vi "Encoder_VI.vi"() -> ()   [LabVIEW 2016]
uses:
  Control 1.ctl
  <vilib>/Instr/_visa.llb/VISA Flush IO Buffer Mask.ctl
  <vilib>/Instr/_visa.llb/VISA Configure Serial Port (Instr).vi
  <vilib>/Utility/file.llb/Write Delimited Spreadsheet (string).vi
panel:
  out "Serial Settings:Number of Bytes at Serial Port":u32
  out "ERRO":dbl
  in  "Limpar":bool
  out "Waveform Graph":waveform(i32)(graph)
  out "Pulso\nInstantâneo":i32
  out "Tempo\nInstantâneo (ms)":u32
  out "iniicio":u32
  in  "Cronômetro para início (s)":string
  out "Identificação":u32
  in  "Endereço":string
  in  "stop":bool
  out "start read":bool
  out "save":bool
  out "start device":bool
  in  "Parar":bool
  out "Configurado Man":bool
  out "Configurado Auto":bool
  out "Desconectado":bool
  out "Conectado":bool
  in  "Frequência \nManual (Hz)":i16
  in  "Frequência \nAutomática (Hz)":u8(ring) items=["50", "100", "200", "500", "1000"]
  in  "Leitura Automática":bool
  in  "Conectar":bool
  in  "salvar dados":bool
  in  "Iniciar dispositivo":bool
  in  "Inicia auto":bool
  in  "Configurar":bool
  in  "Identificar":bool
  in  "Codificar":bool
  out "?":string
  in  "Serial":refnum<visa-resource-name>
  # "Leitura de Encoder - CEFISE"
  # "Status"
  # "Resultado da medida"
  # "Leitura Manual"
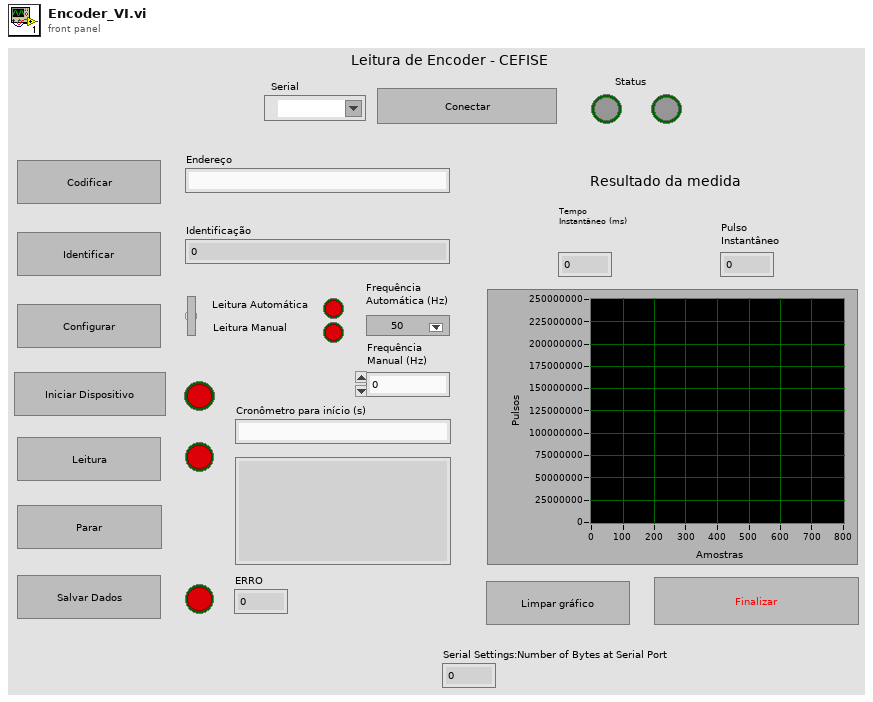
[diagram p1: front panel]
types:
  T1 = typedef "Control 1.ctl" = enum16{"Init", "Wait", "Id", "Codificacao", "Config. Auto", "Config. Man", "Start device", "Read Auto", "Read Again", "Read First", "Stop device", "End", "Save", "erro", "Plot", "Organize", "Limpa"}
  T2 = enum8{"Enabled", "Disabled", "Disabled and Grayed Out"}
  T3 = typedef "VISA Flush IO Buffer Mask.ctl" = u16
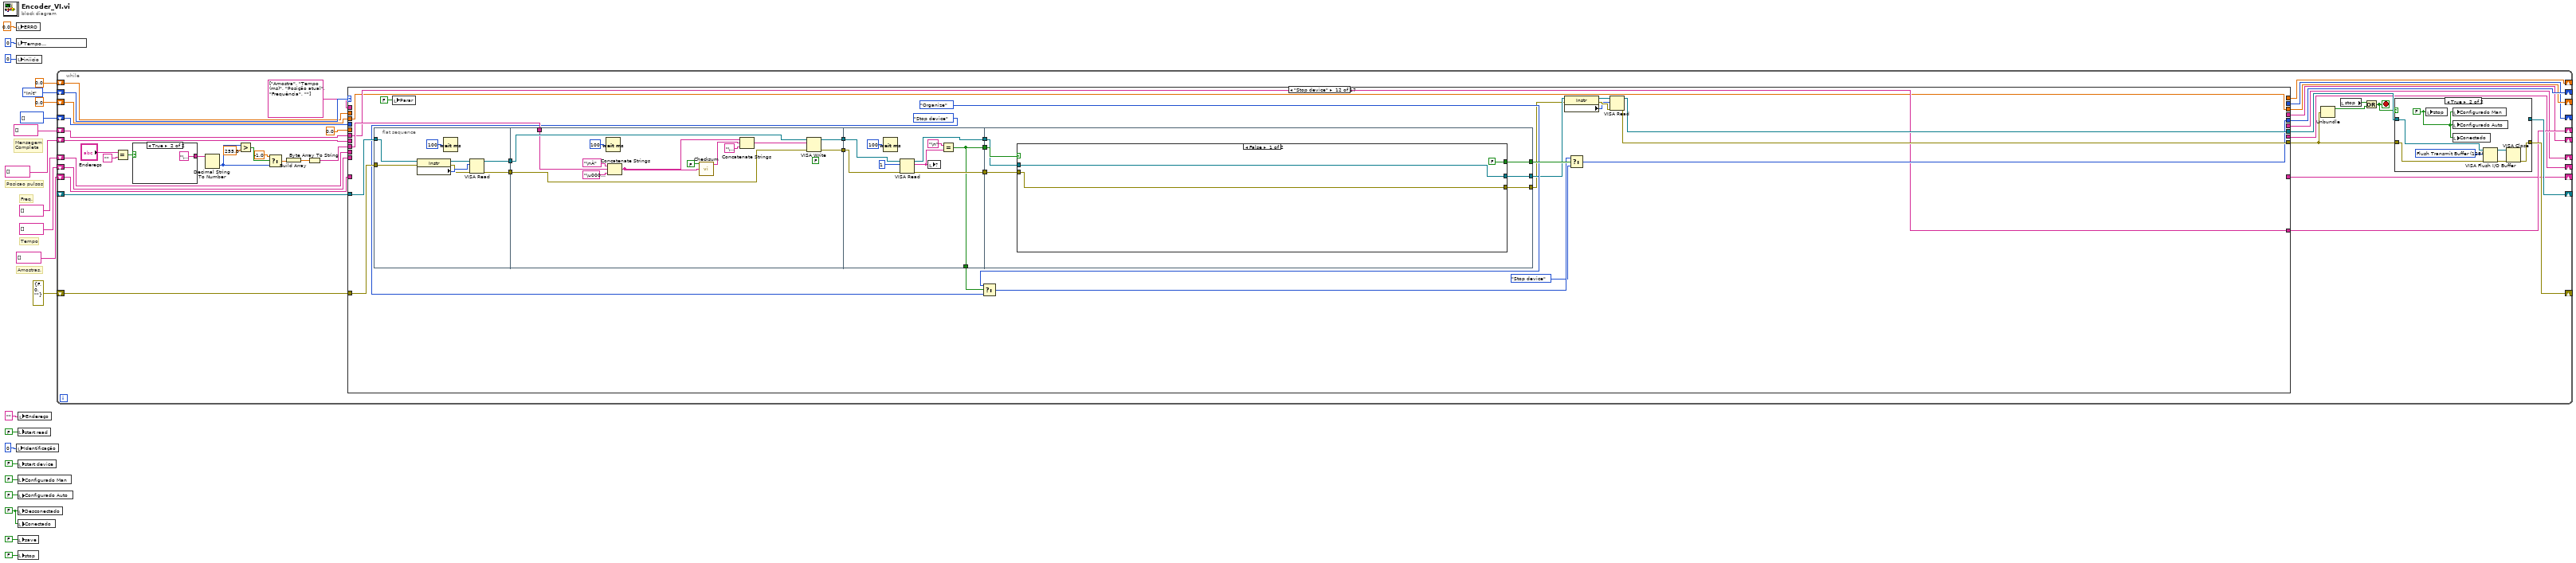
[diagram p0: block diagram]
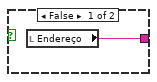
[diagram p2: hidden frame]
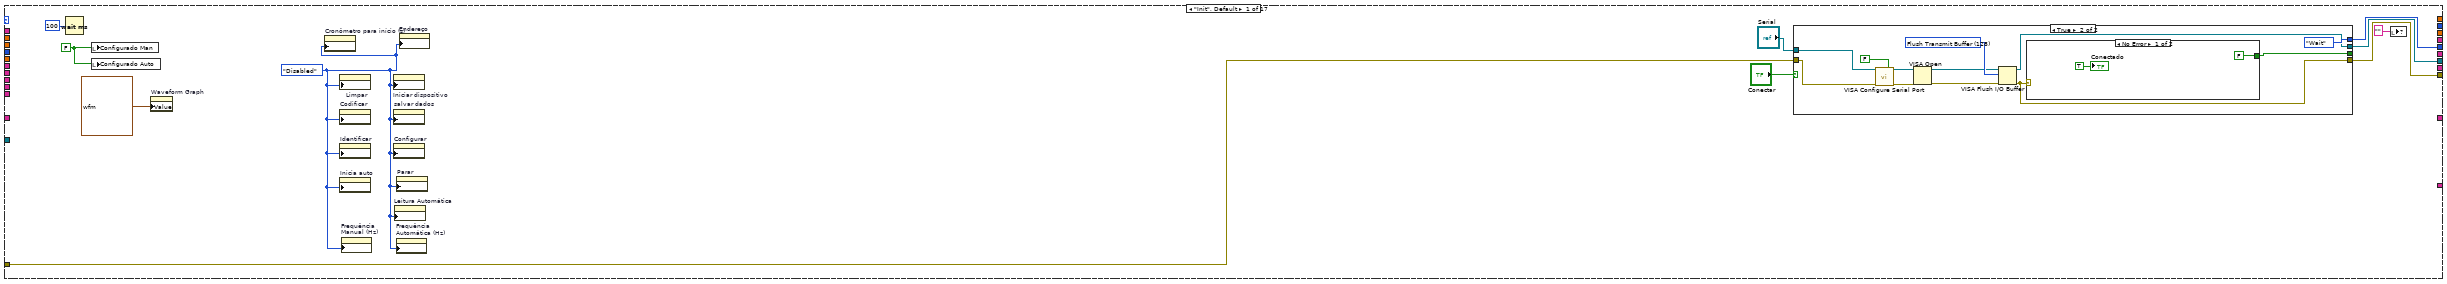
[diagram p4: hidden frame]
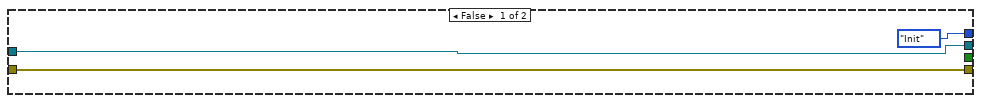
[diagram p5: hidden frame]
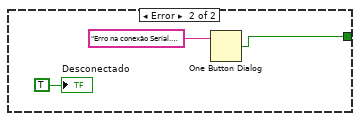
[diagram p6: hidden frame]
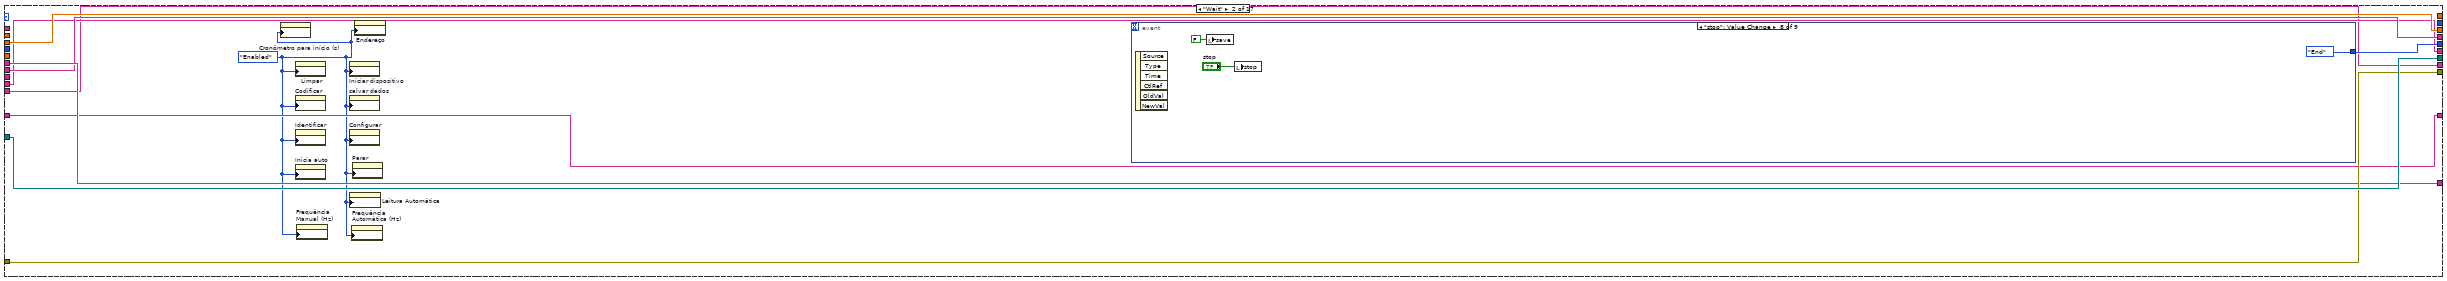
[diagram p7: hidden frame]
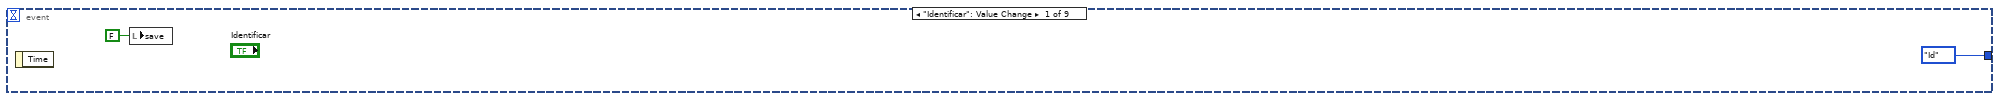
[diagram p8: hidden frame]
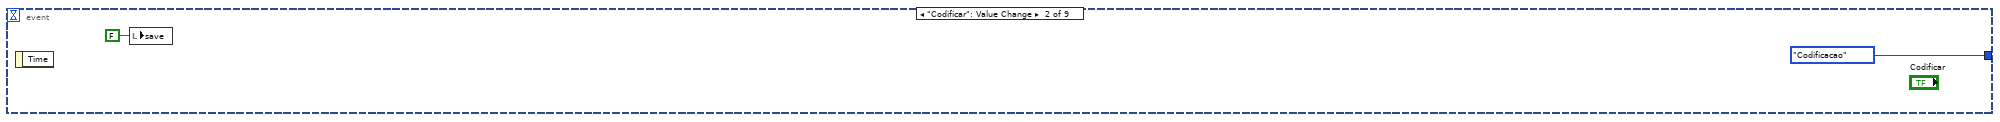
[diagram p9: hidden frame]
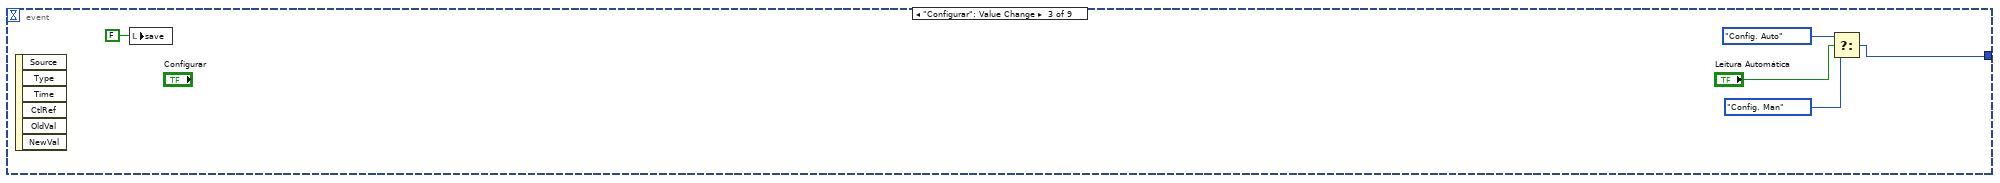
[diagram p10: hidden frame]
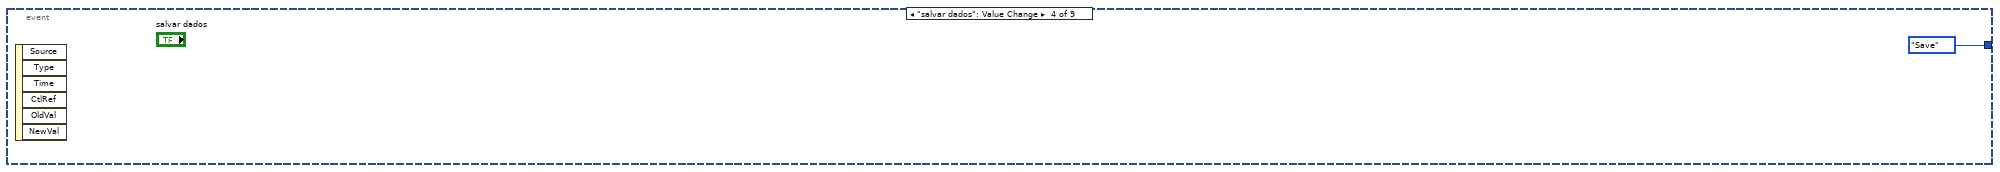
[diagram p11: hidden frame]
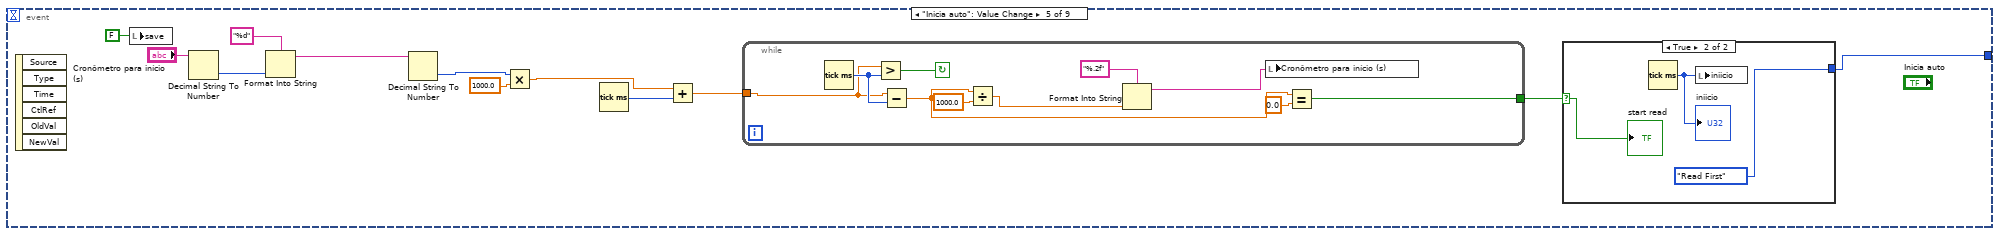
[diagram p12: hidden frame]
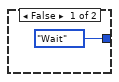
[diagram p13: hidden frame]
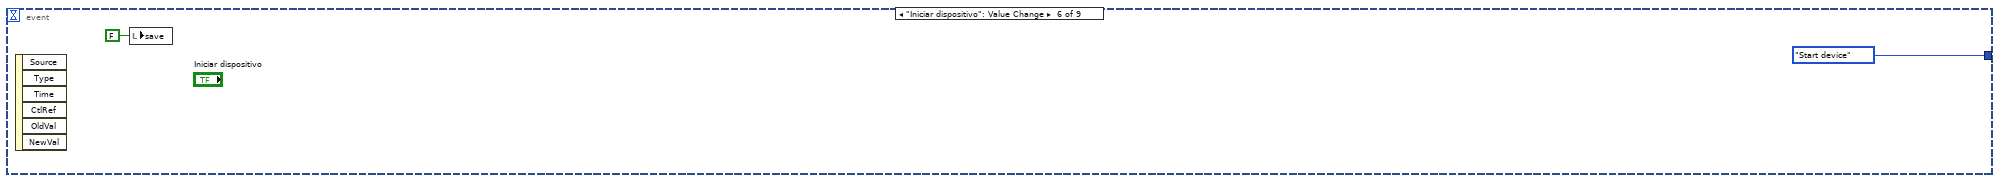
[diagram p14: hidden frame]
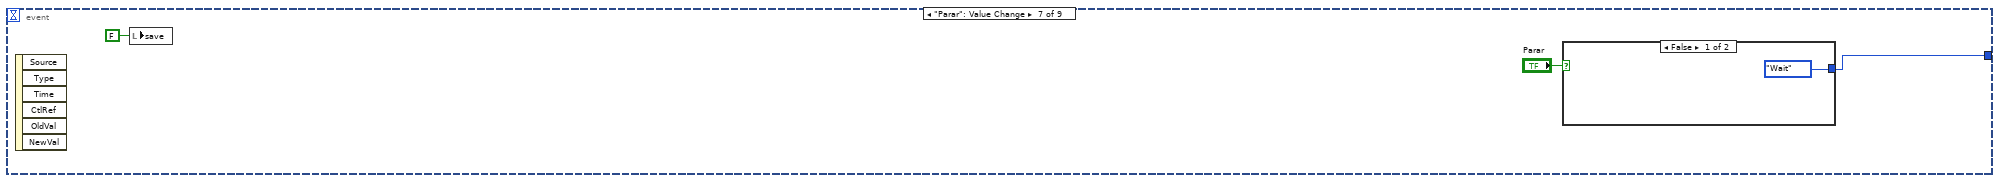
[diagram p15: hidden frame]
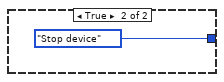
[diagram p16: hidden frame]
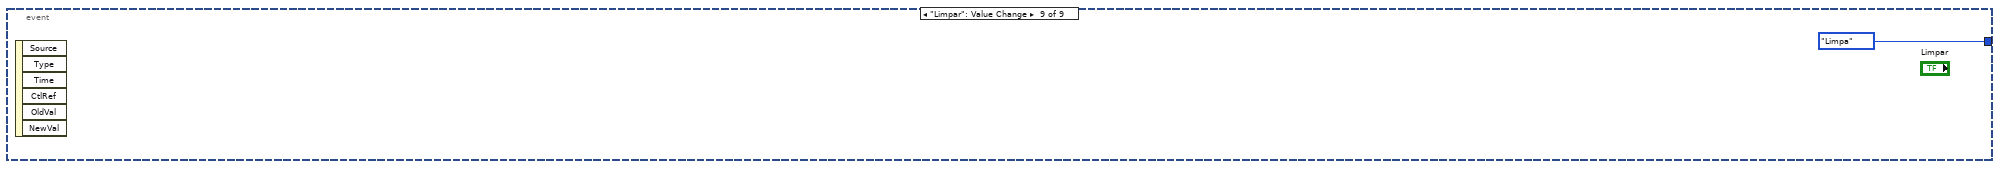
[diagram p17: hidden frame]
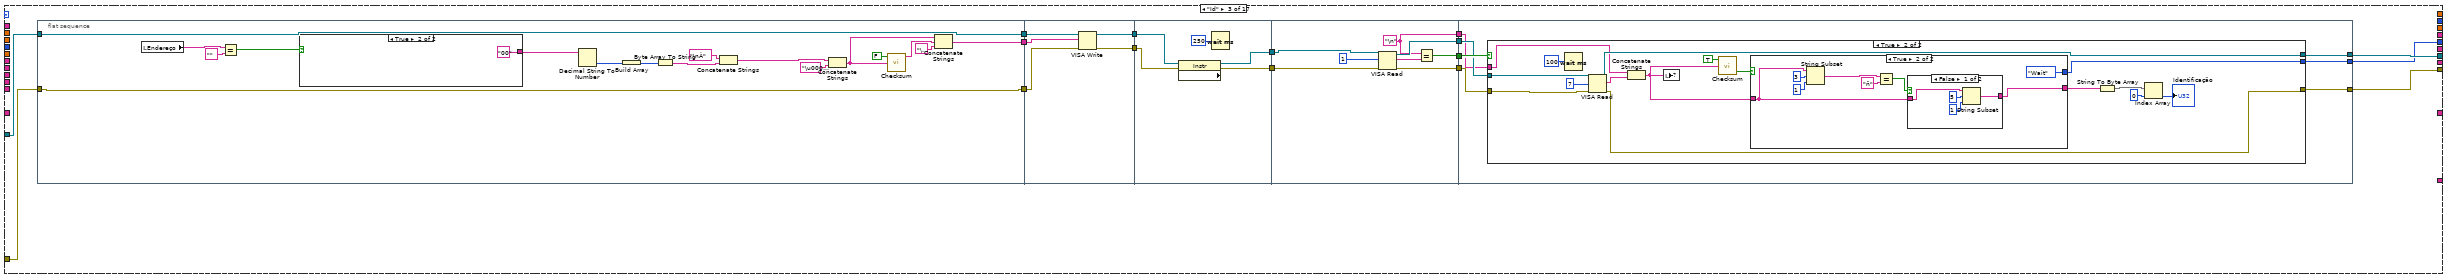
[diagram p18: hidden frame]
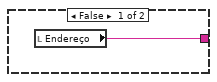
[diagram p19: hidden frame]
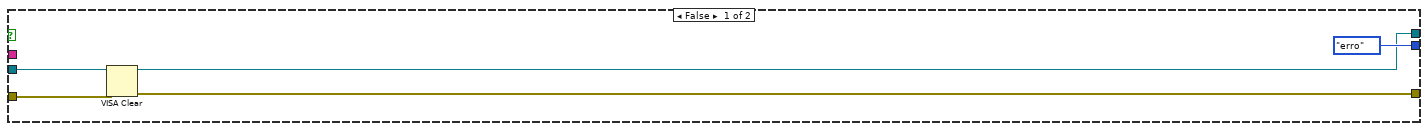
[diagram p20: hidden frame]
diagram:
  w21 = FALSE
  # "Amostras."
  # "Freq."
  # "Tempo"
  # "Posicao pulsos"
  # "Mensagem\nCompleta"
  n1 = local write "ERRO"(0.0 ("ERRO")) -> ()
  n2 = local write "Tempo\nInstantâneo (ms)"(u32 0 ("Recebe")) -> ()
  n3 = local write "iniicio"(u32 0 ("iniicio")) -> ()
  n4 = local write "Identificação"(u32 0 ("Identificação")) -> ()
  n5 = local write "start read"(FALSE ("start read")) -> ()
  n6 = local write "start device"(FALSE ("start device")) -> ()
  n7 = local write "Configurado Man"(FALSE ("Configurado Man")) -> ()
  n8 = local write "Configurado Auto"(FALSE ("Configurado Auto")) -> ()
  n9 = local write "Desconectado"(w21) -> ()
  n10 = local write "Conectado"(w21) -> ()
  n11 = local write "save"(FALSE ("save")) -> ()
  n12 = local write "stop"(FALSE ("save")) -> ()
  n13 = local write "Endereço"("" ("Endereço")) -> ()
  n14 = while {
    shift-right: [w60] -> _
    shift-left: _ -> [w58]
    shift-right: [w59] -> _
    shift-left: errorcluster {"status"=FALSE, "code"=0, "source"=""} ("error in (no error)") -> [w62]
    shift-right: [w57] -> _
    shift-left: Control_1."Init" -> [w56]
    shift-right: [w49] -> _
    shift-left: 0.0 -> [w48]
    shift-right: [w45] -> _
    shift-left: u32[] [] -> [w44]
    shift-right: [w43] -> _
    shift-left: string[] [] -> [w42]
    shift-right: [w33] -> _
    shift-left: string[] [] -> [w32]
    shift-right: [w31] -> _
    shift-left: string[] [] -> [w28]
    shift-right: [w30] -> _
    shift-left: string[] [] -> [w27]
    shift-right: [w29] -> _
    shift-left: string[] [] -> [w26]
    shift-right: [w24] -> _
    shift-left: 0.0 -> [w23]
    stop <- w53 stop-if-true
    n15 = Equal?(x="Endereço", y="" ("write buffer")) -> (x = y?=w51:bool)
    n16 = case shown="True" w51 {
      tunnel: [w63 "\u0000" ("write buffer")] -> w40
      frame False {
        n17 = local read "Endereço"() -> (w63:string)
      }
      frame True {
      }
    }
    n18 = Decimal String To Number(string=w40) -> (number=w36:i32)  [unwired: 2 in, 1 out]
    n19 = Greater?(x=w36, y=255.0 ("x")) -> (0:w39:bool)
    n20 = Select(t=-1.0, s=w39, f=w36) -> (s? t:f=w37:dbl)
    n21 = Build Array(w37) -> (w47:dbl[])
    n22 = Byte Array To String(unsigned byte array=w47) -> (string=w46:string)
    n23 = case shown="\"Stop device\"" w56 {
      tunnel: w58 -> [_ w114 w177 w267 w320 w407 w419 w500 w570 w690 w725 w765 w837 w842 w876 w950 w992]
      tunnel: w62 -> [w84 w113 w176 w266 w321 w408 w418 w499 w571 w689 w724 w764 w836 w841 w875 w951 w991]
      tunnel: [w78 w114 w164 w276 w338 w407 w434 w508 w590 w692 w723 w770 w837 w842 w876 w945 w992] -> w61
      tunnel: [w77 w113 w165 w275 w337 w408 w433 w507 w589 w691 w722 w771 w836 w841 w875 w944 w991] -> w55
      tunnel: [w80 w112 w163 w274 w336 Control_1."Wait" w432 w506 w591 w706 w721 w769 Control_1."Wait" Control_1."Wait" Control_1."Plot" w943 Control_1."Wait"] -> w57
      tunnel: string[] ["Amostra", "Tempo (ms)", "Posição atual", "Frequência", ""] -> [_ _ _ _ _ _ _ _ _ _ _ _ _ w849 _ _ _]
      tunnel: [_ w111 _ _ _ _ w412 _ w579 w695 w720 w766 w833 _ _ _ _] -> w49
      tunnel: w48 -> [_ w111 _ _ _ _ w412 _ w576 w695 w720 w766 w833 _ w873 _ _]
      tunnel: w46 -> [_ _ _ w261 w314 _ w411 w494 _ w694 w719 w768 _ _ _ _ _]
      tunnel: [_ _ _ _ _ _ _ _ w574 _ _ _ _ _ _ _ _] -> w45
      tunnel: w44 -> [_ _ _ _ _ _ _ _ w575 _ w715 _ _ _ _ _ _]
      tunnel: [_ w110 _ _ _ _ _ _ w573 w693 w718 w767 _ _ _ _ _] -> w43
      tunnel: w42 -> [_ w110 _ _ _ _ _ _ w572 w693 w718 w767 _ _ w874 _ _]
      tunnel: w32 -> [_ w109 _ _ _ _ _ _ _ _ _ _ _ w845 w871 _ w990]
      tunnel: w27 -> [_ w107 _ _ _ _ _ _ _ _ _ _ _ w838 w865 _ w989]
      tunnel: w28 -> [_ w108 _ _ _ _ _ _ _ _ _ _ _ w839 w866 _ w988]
      tunnel: w26 -> [_ w106 _ _ _ _ _ _ _ _ _ _ _ w840 w864 _ w987]
      tunnel: [_ w109 _ _ _ _ _ _ _ _ _ _ _ _ w872 _ w990] -> w33
      tunnel: [_ w108 _ _ _ _ _ _ _ _ _ _ _ _ w870 _ w988] -> w31
      tunnel: [_ w107 _ _ _ _ _ _ _ _ _ _ _ _ w869 _ w989] -> w30
      tunnel: [_ w106 _ _ _ _ _ _ _ _ _ _ _ _ w868 _ w987] -> w29
      tunnel: 0.0 -> [_ _ _ _ _ _ _ _ _ _ _ _ _ _ w867 _ _]
      tunnel: [_ _ _ _ _ _ _ _ w566 w688 w713 _ _ _ _ _ _] -> w24
      tunnel: w23 -> [_ _ _ _ _ _ _ _ w565 w688 w713 _ _ _ _ _ _]
      frame "Init", Default {
        w74 = T2."Disabled" ("Disabled")
        w81 = FALSE ("Configurado Man")
        n24 = Wait (ms)(milliseconds to wait=u32 100) -> ()  [unwired: 1 out]
        n25 = local write "Configurado Man"(w81) -> ()
        n26 = local write "Configurado Auto"(w81) -> ()
        n27 = property on="Waveform Graph" class="WFGraph (strict)"("Value"=waveform(i32) {"t0"=timestamp(0 s since 1904-01-01), "dt"=0.0, "Y"=[]} ("Waveform Graph")) -> ()  [unwired: 2 in, 2 out]
        n28 = property on="Cronômetro para início (s)" class="Str"("DisabledEnum"=w74) -> ()  [unwired: 2 in, 2 out]
        n29 = property on="Limpar" class="Bool"("DisabledEnum"=w74) -> ()  [unwired: 2 in, 2 out]
        n30 = property on="Codificar" class="Bool"("DisabledEnum"=w74) -> ()  [unwired: 2 in, 2 out]
        n31 = property on="Identificar" class="Bool"("DisabledEnum"=w74) -> ()  [unwired: 2 in, 2 out]
        n32 = property on="Inicia auto" class="Bool"("DisabledEnum"=w74) -> ()  [unwired: 2 in, 2 out]
        n33 = property on="Frequência \nManual (Hz)" class="DigNum (strict)"("DisabledEnum"=w74) -> ()  [unwired: 2 in, 2 out]
        n34 = property on="Iniciar dispositivo" class="Bool"("DisabledEnum"=w74) -> ()  [unwired: 2 in, 2 out]
        n35 = property on="salvar dados" class="Bool"("DisabledEnum"=w74) -> ()  [unwired: 2 in, 2 out]
        n36 = property on="Configurar" class="Bool"("DisabledEnum"=w74) -> ()  [unwired: 2 in, 2 out]
        n37 = property on="Leitura Automática" class="Bool (strict)"("DisabledEnum"=w74) -> ()  [unwired: 2 in, 2 out]
        n38 = property on="Frequência \nAutomática (Hz)" class="Ring (strict)"("DisabledEnum"=w74) -> ()  [unwired: 2 in, 2 out]
        n39 = property on="Parar" class="Bool (strict)"("DisabledEnum"=w74) -> ()  [unwired: 2 in, 2 out]
        n40 = property on="Endereço" class="Str"("DisabledEnum"=w74) -> ()  [unwired: 2 in, 2 out]
        n41 = case shown="True" "Conectar" {
          tunnel: "Serial" -> [w86 w90]
          tunnel: w84 -> [w85 w89]
          tunnel: [Control_1."Init" Control_1."Wait"] -> w80
          tunnel: [w86 w94] -> w78
          tunnel: [w85 w93] -> w77
          tunnel: [_ w95] -> _
          frame False {
          }
          frame True {
            w99 = T3 128 items=["Flush Receive Buffer"=16, "Write Transmit Buffer to Device"=32, "Flush Receive Buffer (No I/O)"=64, "Flush Transmit Buffer"=128] ("Mask")
            n42 = call-poly "VISA Configure Serial Port"("VISA resource name"=w90, "Enable Termination\nChar (T)"=FALSE ("Enable Termination\nChar (T)"), "error in (no error)"=w89) -> ("VISA resource name out"=w92:refnum<visa-resource-name>, "error out"=w91:errorcluster)  [unwired: 11 in]
            n43 = VISA Open(error in (no error)=w91, VISA resource name=w92) -> (VISA resource name=w97:refnum<visa-resource-name>, error out=w98:errorcluster)  [unwired: 3 in]
            n44 = VISA Flush I/O Buffer(VISA resource name=w97, mask (16)=w99, error in (no error)=w98) -> (VISA resource name out=w94:refnum<visa-resource-name>, error out=w93:errorcluster)
            n45 = case shown="No Error" w93 {
              tunnel: [FALSE ("true") w102] -> w95
              frame No Error {
                "Conectado" <- TRUE ("Conectado")
              }
              frame Error {
                n46 = One Button Dialog(message="Erro na conexão Serial. Verifique as ligações e reinicie o programa.") -> (true=w102:bool)  [unwired: 1 in]
                "Desconectado" <- TRUE ("Desconectado")
              }
            }
          }
        }
        n47 = local write item#1("") -> ()
      }
      frame "Wait" {
        w105 = T2."Enabled" ("Disabled")
        n48 = property on="Cronômetro para início (s)" class="Str"("DisabledEnum"=w105) -> ()  [unwired: 2 in, 2 out]
        n49 = property on="Limpar" class="Bool"("DisabledEnum"=w105) -> ()  [unwired: 2 in, 2 out]
        n50 = property on="Codificar" class="Bool"("DisabledEnum"=w105) -> ()  [unwired: 2 in, 2 out]
        n51 = property on="Identificar" class="Bool"("DisabledEnum"=w105) -> ()  [unwired: 2 in, 2 out]
        n52 = property on="Inicia auto" class="Bool"("DisabledEnum"=w105) -> ()  [unwired: 2 in, 2 out]
        n53 = property on="Frequência \nManual (Hz)" class="DigNum (strict)"("DisabledEnum"=w105) -> ()  [unwired: 2 in, 2 out]
        n54 = property on="Iniciar dispositivo" class="Bool"("DisabledEnum"=w105) -> ()  [unwired: 2 in, 2 out]
        n55 = property on="salvar dados" class="Bool"("DisabledEnum"=w105) -> ()  [unwired: 2 in, 2 out]
        n56 = property on="Configurar" class="Bool"("DisabledEnum"=w105) -> ()  [unwired: 2 in, 2 out]
        n57 = property on="Leitura Automática" class="Bool (strict)"("DisabledEnum"=w105) -> ()  [unwired: 2 in, 2 out]
        n58 = property on="Frequência \nAutomática (Hz)" class="Ring (strict)"("DisabledEnum"=w105) -> ()  [unwired: 2 in, 2 out]
        n59 = property on="Parar" class="Bool (strict)"("DisabledEnum"=w105) -> ()  [unwired: 2 in, 2 out]
        n60 = property on="Endereço" class="Str"("DisabledEnum"=w105) -> ()  [unwired: 2 in, 2 out]
        n61 = event shown="[7] \"stop\": Value Change" {
          selector: _ -> [_ _ _ _ _ _ _ _ _]
          dyn-events: _ -> [_ _ _ _ _ _ _ _ _]
          timeout: _ -> [_ _ _ _ _ _ _ _ _]
          tunnel: [Control_1."Id" Control_1."Codificacao" w120 Control_1."Save" w136 Control_1."Start device" w155 Control_1."End" Control_1."Limpa"] -> w112
          event "Identificar": Value Change {
            n62 = event-data() -> ()  [unwired: 1 in, 1 out]
            n63 = local write "save"(FALSE ("salvar dados")) -> ()
          }
          event "Codificar": Value Change {
            n64 = event-data() -> ()  [unwired: 1 in, 1 out]
            n65 = local write "save"(FALSE ("salvar dados")) -> ()
          }
          event "Configurar": Value Change {
            n66 = event-data() -> ()  [unwired: 1 in, 6 out]
            n67 = local write "save"(FALSE ("salvar dados")) -> ()
            n68 = Select(t=Control_1."Config. Auto", s="Leitura Automática", f=Control_1."Config. Man") -> (s? t:f=w120:T1)
          }
          event "salvar dados": Value Change {
            n69 = event-data() -> ()  [unwired: 1 in, 6 out]
          }
          event "Inicia auto": Value Change {
            n70 = event-data() -> ()  [unwired: 1 in, 6 out]
            n71 = local write "save"(FALSE ("salvar dados")) -> ()
            n72 = Decimal String To Number(string="Cronômetro para início (s)") -> (number=w132:i32)  [unwired: 2 in, 1 out]
            n73 = Format Into String(format string="%d", w132) -> (resulting string=w133:string)  [unwired: 2 in, 1 out]
            n74 = Decimal String To Number(string=w133) -> (number=w134:i32)  [unwired: 2 in, 1 out]
            n75 = Multiply(x=w134, y=1000.0) -> (x*y=w129:dbl)
            n76 = Tick Count (ms)() -> (millisecond timer value=w130:u32)
            n77 = Add(x=w129, y=w130) -> (x+y=w126:dbl)
            n78 = while {
              tunnel: [w137] -> w135
              tunnel: w126 -> [w139]
              stop <- w138 continue-if-true
              n79 = Tick Count (ms)() -> (millisecond timer value=w140:u32)
              n80 = Greater?(x=w139, y=w140) -> (0:w138:bool)
              n81 = Subtract(x=w139, y=w140) -> (x-y=w144:dbl)
              n82 = Divide(x=w144, y=1000.0) -> (x/y=w146:dbl)
              n83 = Format Into String(format string="%.2f", w146) -> (resulting string=w143:string)  [unwired: 2 in, 1 out]
              n84 = local write "Cronômetro para início (s)"(w143) -> ()
              n85 = Equal?(x=w144, y=0.0) -> (x = y?=w137:bool)
            }
            n86 = case shown="True" w135 {
              selector: w135 -> [_ w149]
              tunnel: [Control_1."Wait" Control_1."Read First"] -> w136
              frame False {
              }
              frame True {
                n87 = Tick Count (ms)() -> (millisecond timer value=w148:u32)
                "iniicio" <- w148
                n88 = local write "iniicio"(w148) -> ()
                "start read" <- w149
              }
            }
          }
          event "Iniciar dispositivo": Value Change {
            n89 = event-data() -> ()  [unwired: 1 in, 6 out]
            n90 = local write "save"(FALSE ("salvar dados")) -> ()
          }
          event "Parar": Value Change {
            n91 = event-data() -> ()  [unwired: 1 in, 6 out]
            n92 = local write "save"(FALSE ("salvar dados")) -> ()
            n93 = case shown="False" "Parar" {
              tunnel: [Control_1."Wait" Control_1."Stop device"] -> w155
              frame False {
              }
              frame True {
              }
            }
          }
          event "stop": Value Change {
            n94 = event-data() -> ()  [unwired: 1 in, 6 out]
            n95 = local write "save"(FALSE ("salvar dados")) -> ()
            n96 = local write "stop"("stop") -> ()
          }
          event "Limpar": Value Change {
            n97 = event-data() -> ()  [unwired: 1 in, 6 out]
          }
        }
      }
      frame "Id" {
        n98 = flat-sequence {
          tunnel: w176 -> [w193]
          tunnel: w177 -> [w194]
          tunnel: [w194] -> w173
          tunnel: [w193] -> w172
          tunnel: [w186] -> w171
          tunnel: [w199] -> w175
          tunnel: [w198] -> w174
          tunnel: w173 -> [w201]
          tunnel: w172 -> [w200]
          tunnel: w171 -> [w197]
          tunnel: w175 -> [w206]
          tunnel: w174 -> [w205]
          tunnel: [w204] -> w170
          tunnel: [w203] -> w169
          tunnel: w170 -> [w213]
          tunnel: w169 -> [w214]
          tunnel: [w210] -> w168
          tunnel: [w209] -> w167
          tunnel: [w208] -> w166
          tunnel: [w207] -> w162
          tunnel: w168 -> [w221]
          tunnel: w167 -> [w220]
          tunnel: w166 -> [w219]
          tunnel: [w218] -> w165
          tunnel: [w217] -> w164
          tunnel: [w216] -> w163
          tunnel: w162 -> [w215]
          frame #0 {
            n99 = local read "Endereço"() -> (w185:string)
            n100 = Equal?(x=w185, y="") -> (x = y?=w183:bool)
            n101 = case shown="True" w183 {
              tunnel: [w195 "00" ("string")] -> w178
              frame False {
                n102 = local read "Endereço"() -> (w195:string)
              }
              frame True {
              }
            }
            n103 = Decimal String To Number(string=w178) -> (number=w180:i32)  [unwired: 2 in, 1 out]
            n104 = Build Array(w180) -> (w181:i32[])
            n105 = Byte Array To String(unsigned byte array=w181) -> (string=w179:string)
            n106 = Concatenate Strings("\nÀ" ("write buffer"), w179) -> (w191:string)
            n107 = Concatenate Strings(w191, "\u0001\u0000" ("string")) -> (w188:string)
            n108 = call "Checksum.vi"("String"=w188, "Check soma?"=FALSE) -> ("Check"=w189:string)  [unwired: 1 in, 2 out]
            n109 = Concatenate Strings(w188, w189, "\u000f" ("string")) -> (w186:string)
          }
          frame #1 {
            n110 = VISA Write(VISA resource name=w201, write buffer=w197, error in (no error)=w200) -> (VISA resource name out=w199:refnum<visa-resource-name>, error out=w198:errorcluster)  [unwired: 1 out]
          }
          frame #2 {
            n111 = property class="Instr" props=["Serial Settings:Number of Bytes at Serial Port"](reference=w206, error in=w205) -> (reference out=w204:refnum<visa-resource-name>, error out=w203:errorcluster)  [unwired: 1 out]
            n112 = Wait (ms)(milliseconds to wait=u32 250) -> ()  [unwired: 1 out]
          }
          frame #3 {
            w207 = "\n" ("x")
            n113 = VISA Read(VISA resource name=w213, byte count=u32 1, error in (no error)=w214) -> (VISA resource name out=w208:refnum<visa-resource-name>, read buffer=w211:string, error out=w209:errorcluster)  [unwired: 1 out]
            n114 = Equal?(x=w207, y=w211) -> (x = y?=w210:bool)
          }
          frame #4 {
            n115 = case shown="True" w221 {
              tunnel: w220 -> [w222 w239]
              tunnel: w219 -> [w225 w238]
              tunnel: [w224 w232] -> w217
              tunnel: [w223 w231] -> w218
              tunnel: [Control_1."erro" w228] -> w216
              tunnel: w215 -> [_ w229]
              frame False {
                n116 = VISA Clear(VISA resource name=w225, error in (no error)=w222) -> (VISA resource name out=w224:refnum<visa-resource-name>, error out=w223:errorcluster)
              }
              frame True {
                n117 = Wait (ms)(milliseconds to wait=u32 100) -> ()  [unwired: 1 out]
                n118 = VISA Read(VISA resource name=w238, byte count=u32 7, error in (no error)=w239) -> (VISA resource name out=w232:refnum<visa-resource-name>, read buffer=w230:string, error out=w231:errorcluster)  [unwired: 1 out]
                n119 = Concatenate Strings(w229, w230) -> (w227:string)
                n120 = local write item#1(w227) -> ()
                n121 = call "Checksum.vi"("String"=w227, "Check soma?"=TRUE) -> ("Checksum?"=w233:bool)  [unwired: 1 in, 2 out]
                n122 = case shown="True" w233 {
                  tunnel: ["\u0000" ("read buffer") w252] -> w237
                  tunnel: w227 -> [_ w245]
                  tunnel: [Control_1."erro" Control_1."Wait"] -> w228
                  frame False {
                  }
                  frame True {
                    n123 = String Subset(string=w245, offset (0)=3, length (rest)=1 ("length (rest)")) -> (substring=w248:string)
                    n124 = Equal?(x=w248, y="ñ") -> (x = y?=w246:bool)
                    n125 = case shown="False" w246 {
                      tunnel: [w253 w258] -> w252
                      tunnel: w245 -> [w254 w257]
                      frame False {
                        n126 = String Subset(string=w254, offset (0)=5, length (rest)=1 ("length (rest)")) -> (substring=w253:string)
                      }
                      frame True {
                        n127 = String Subset(string=w257, offset (0)=1, length (rest)=1 ("length (rest)")) -> (substring=w258:string)
                      }
                    }
                  }
                }
                n128 = String To Byte Array(string=w237) -> (unsigned byte array=w236:u8[])
                n129 = Index Array(array=w236, index=0 ("length")) -> (element=→"Identificação":u8)
              }
            }
          }
        }
      }
      frame "Codificacao" {
        n130 = Concatenate Strings("\nÀ" ("write buffer"), w261, "\u0001\u0001" ("write buffer"), w261) -> (w269:string)
        n131 = call "Checksum.vi"("String"=w269, "Check soma?"=FALSE) -> ("Checksum?"=w263:bool, "Check"=w270:string)  [unwired: 1 in, 1 out]
        n132 = Concatenate Strings(w269, w270, "\u000f" ("write buffer")) -> (w271:string)
        n133 = VISA Write(VISA resource name=w267, write buffer=w271, error in (no error)=w266) -> (VISA resource name out=w264:refnum<visa-resource-name>, error out=w265:errorcluster)  [unwired: 1 out]
        n134 = case shown="True" w263 {
          tunnel: [w278 w284] -> w276
          tunnel: [w277 w283] -> w275
          tunnel: [Control_1."erro" Control_1."Wait"] -> w274
          tunnel: w265 -> [w277 w282]
          tunnel: w264 -> [w278 w281]
          frame False {
          }
          frame True {
            n135 = flat-sequence {
              tunnel: [w295] -> w290
              tunnel: [w294] -> w289
              tunnel: w282 -> [w292]
              tunnel: w281 -> [w291]
              tunnel: w290 -> [w303]
              tunnel: w289 -> [w302]
              tunnel: [w301] -> w288
              tunnel: [w300] -> w287
              tunnel: [w298] -> w286
              tunnel: [w297] -> w285
              tunnel: [w307] -> w284
              tunnel: w288 -> [w307]
              tunnel: [w306] -> w283
              tunnel: w287 -> [w306]
              tunnel: w286 -> [w305]
              tunnel: w285 -> [w304]
              frame #0 {
                n136 = property class="Instr" props=["Serial Settings:Number of Bytes at Serial Port"](reference=w291, error in=w292) -> (reference out=w295:refnum<visa-resource-name>, error out=w294:errorcluster)  [unwired: 1 out]
                n137 = Wait (ms)(milliseconds to wait=u32 10) -> ()  [unwired: 1 out]
              }
              frame #1 {
                n138 = VISA Read(VISA resource name=w303, byte count=u32 8, error in (no error)=w302) -> (VISA resource name out=w301:refnum<visa-resource-name>, read buffer=w297:string, error out=w300:errorcluster)  [unwired: 1 out]
                n139 = local write item#1(w297) -> ()
                n140 = call "Checksum.vi"("String"=w297, "Check soma?"=TRUE) -> ("Checksum?"=w298:bool)  [unwired: 1 in, 2 out]
              }
              frame #2 {
                n141 = case shown="True" w305 {
                  tunnel: w304 -> [_ w312]
                  tunnel: ["\u0000" ("read buffer") w309] -> _
                  frame False {
                  }
                  frame True {
                    n142 = String Subset(string=w312, offset (0)=5, length (rest)=1 ("length (rest)")) -> (substring=w309:string)
                  }
                }
              }
            }
          }
        }
      }
      frame "Config. Auto" {
        n143 = property on="Frequência \nAutomática (Hz)" class="Ring (strict)"() -> ("RingText.Text"=w330:string)  [unwired: 2 in, 2 out]
        n144 = Decimal String To Number(string=w330) -> (number=w328:i32)  [unwired: 2 in, 1 out]
        n145 = Reciprocal(x=w328) -> (1/x=w327:dbl)
        n146 = Multiply(x=1000, y=w327) -> (x*y=w325:dbl)
        n147 = Format Into String(format string="%d", w325) -> (resulting string=w333:string)  [unwired: 2 in, 1 out]
        n148 = Decimal String To Number(string=w333) -> (number=w313:i32)  [unwired: 2 in, 1 out]
        n149 = Build Array(w313) -> (w331:i32[])
        n150 = Byte Array To String(unsigned byte array=w331) -> (string=w329:string)
        n151 = Concatenate Strings("\nÀ" ("write buffer"), w314, "\u0002\u0002\u0001" ("write buffer"), w329) -> (w319:string)
        n152 = call "Checksum.vi"("String"=w319, "Check soma?"=FALSE) -> ("Checksum?"=w318:bool, "Check"=w316:string)  [unwired: 1 in, 1 out]
        n153 = Concatenate Strings(w319, w316, "\u000f" ("string")) -> (w334:string)
        n154 = VISA Write(VISA resource name=w320, write buffer=w334, error in (no error)=w321) -> (VISA resource name out=w323:refnum<visa-resource-name>, error out=w322:errorcluster)  [unwired: 1 out]
        n155 = case shown="True" w318 {
          tunnel: [w340 w346] -> w338
          tunnel: [w339 w345] -> w337
          tunnel: [Control_1."erro" Control_1."Wait"] -> w336
          tunnel: w323 -> [w340 w344]
          tunnel: w322 -> [w339 w343]
          frame False {
          }
          frame True {
            n156 = flat-sequence {
              tunnel: [w360] -> w355
              tunnel: [w359] -> w354
              tunnel: w344 -> [w357]
              tunnel: w343 -> [w356]
              tunnel: w355 -> [w368]
              tunnel: [w365] -> w353
              tunnel: w354 -> [w367]
              tunnel: [w364] -> w352
              tunnel: [w362] -> w351
              tunnel: [w361] -> w350
              tunnel: w353 -> [w372]
              tunnel: [w374] -> w349
              tunnel: [w375] -> w348
              tunnel: [w373] -> w347
              tunnel: w352 -> [w371]
              tunnel: w351 -> [w370]
              tunnel: w350 -> [w369]
              tunnel: [w392] -> w345
              tunnel: [w393] -> w346
              tunnel: w349 -> [w395]
              tunnel: w348 -> [w394]
              tunnel: w347 -> [w396]
              frame #0 {
                n157 = property class="Instr" props=["Serial Settings:Number of Bytes at Serial Port"](reference=w357, error in=w356) -> (reference out=w360:refnum<visa-resource-name>, error out=w359:errorcluster)  [unwired: 1 out]
                n158 = Wait (ms)(milliseconds to wait=u32 100) -> ()  [unwired: 1 out]
              }
              frame #1 {
                w361 = "\n" ("x")
                n159 = VISA Read(VISA resource name=w368, byte count=u32 1, error in (no error)=w367) -> (VISA resource name out=w365:refnum<visa-resource-name>, read buffer=w363:string, error out=w364:errorcluster)  [unwired: 1 out]
                n160 = Equal?(x=w361, y=w363) -> (x = y?=w362:bool)
              }
              frame #2 {
                n161 = case shown="True" w370 {
                  tunnel: [w377 w391] -> w375
                  tunnel: [w378 w390] -> w374
                  tunnel: [FALSE ("Checksum?") w389] -> w373
                  tunnel: w372 -> [w380 w387]
                  tunnel: w371 -> [w379 w386]
                  tunnel: w369 -> [_ w383]
                  frame False {
                    w381 = T3 16 items=["Flush Receive Buffer"=16, "Write Transmit Buffer to Device"=32, "Flush Receive Buffer (No I/O)"=64, "Flush Transmit Buffer"=128] ("Mask")
                    n162 = VISA Flush I/O Buffer(VISA resource name=w380, mask (16)=w381, error in (no error)=w379) -> (VISA resource name out=w378:refnum<visa-resource-name>, error out=w377:errorcluster)
                  }
                  frame True {
                    n163 = VISA Read(VISA resource name=w387, byte count=u32 6, error in (no error)=w386) -> (VISA resource name out=w390:refnum<visa-resource-name>, read buffer=w384:string, error out=w391:errorcluster)  [unwired: 1 out]
                    n164 = Concatenate Strings(w383, w384) -> (w382:string)
                    n165 = local write item#1(w382) -> ()
                    n166 = call "Checksum.vi"("String"=w382, "Check soma?"=TRUE) -> ("Checksum?"=w389:bool)  [unwired: 1 in, 2 out]
                  }
                }
              }
              frame #3 {
                n167 = case shown="False" w396 {
                  tunnel: w396 -> [_ w405]
                  tunnel: w395 -> [w401 w403]
                  tunnel: w394 -> [w400 w402]
                  tunnel: [w399 w403] -> w393
                  tunnel: [w398 w402] -> w392
                  frame False {
                    w397 = T3 16 items=["Flush Receive Buffer"=16, "Write Transmit Buffer to Device"=32, "Flush Receive Buffer (No I/O)"=64, "Flush Transmit Buffer"=128] ("Mask")
                    n168 = VISA Flush I/O Buffer(VISA resource name=w401, mask (16)=w397, error in (no error)=w400) -> (VISA resource name out=w399:refnum<visa-resource-name>, error out=w398:errorcluster)
                  }
                  frame True {
                    n169 = local write "Configurado Auto"(w405) -> ()
                    n170 = local write "Configurado Man"(FALSE ("Configurado Man")) -> ()
                    "Configurado Auto" <- w405
                  }
                }
              }
            }
          }
        }
      }
      frame "Limpa" {
        n171 = property on="Waveform Graph" class="WFGraph (strict)"("Value"=waveform(i32) {"t0"=timestamp(0 s since 1904-01-01), "dt"=0.0, "Y"=[]} ("Waveform Graph")) -> ()  [unwired: 2 in, 2 out]
      }
      frame "Config. Man" {
        n172 = local write "Frequência \nManual (Hz)"("Frequência \nManual (Hz)") -> ()
        n173 = Reciprocal(x="Frequência \nManual (Hz)") -> (1/x=w416:dbl)
        n174 = Multiply(x=1000, y=w416) -> (x*y=w414:dbl)
        n175 = Format Into String(w414) -> (resulting string=w417:string)  [unwired: 3 in, 1 out]
        n176 = Decimal String To Number(string=w417) -> (number=w413:i32)  [unwired: 2 in, 1 out]
        n177 = Build Array(w413) -> (w426:i32[])
        n178 = Byte Array To String(unsigned byte array=w426) -> (string=w425:string)
        n179 = Concatenate Strings("\nÀ" ("write buffer"), w411, "\u0002\u0002\u0002" ("write buffer"), w425) -> (w427:string)
        n180 = call "Checksum.vi"("String"=w427, "Check soma?"=FALSE) -> ("Checksum?"=w420:bool, "Check"=w430:string)  [unwired: 1 in, 1 out]
        n181 = Concatenate Strings(w427, w430, "\u000f" ("write buffer")) -> (w428:string)
        n182 = VISA Write(VISA resource name=w419, write buffer=w428, error in (no error)=w418) -> (VISA resource name out=w423:refnum<visa-resource-name>, error out=w422:errorcluster)  [unwired: 1 out]
        n183 = case shown="True" w420 {
          tunnel: [w436 w442] -> w434
          tunnel: [w435 w441] -> w433
          tunnel: [Control_1."erro" Control_1."Wait"] -> w432
          tunnel: w423 -> [w436 w439]
          tunnel: w422 -> [w435 w438]
          frame False {
          }
          frame True {
            n184 = flat-sequence {
              tunnel: [w455] -> w451
              tunnel: [w454] -> w450
              tunnel: w439 -> [w453]
              tunnel: w438 -> [w452]
              tunnel: w451 -> [w464]
              tunnel: [w462] -> w449
              tunnel: w450 -> [w463]
              tunnel: [w461] -> w448
              tunnel: [w458] -> w447
              tunnel: [w457] -> w446
              tunnel: [w471] -> w445
              tunnel: [w470] -> w444
              tunnel: [w469] -> w443
              tunnel: w449 -> [w468]
              tunnel: w448 -> [w467]
              tunnel: w447 -> [w466]
              tunnel: w446 -> [w465]
              tunnel: [w489] -> w441
              tunnel: [w490] -> w442
              tunnel: w445 -> [w490]
              tunnel: w444 -> [w489]
              tunnel: w443 -> [w488]
              frame #0 {
                n185 = property class="Instr" props=["Serial Settings:Number of Bytes at Serial Port"](reference=w453, error in=w452) -> (reference out=w455:refnum<visa-resource-name>, error out=w454:errorcluster)  [unwired: 1 out]
                n186 = Wait (ms)(milliseconds to wait=u32 10) -> ()  [unwired: 1 out]
              }
              frame #1 {
                w457 = "\n" ("x")
                n187 = VISA Read(VISA resource name=w464, byte count=u32 1, error in (no error)=w463) -> (VISA resource name out=w462:refnum<visa-resource-name>, read buffer=w460:string, error out=w461:errorcluster)  [unwired: 1 out]
                n188 = Equal?(x=w457, y=w460) -> (x = y?=w458:bool)
              }
              frame #2 {
                n189 = case shown="True" w466 {
                  tunnel: [w474 w486] -> w471
                  tunnel: [w473 w485] -> w470
                  tunnel: [FALSE ("Checksum?") w484] -> w469
                  tunnel: w468 -> [w476 w483]
                  tunnel: w467 -> [w475 w482]
                  tunnel: w465 -> [_ w479]
                  frame False {
                    n190 = VISA Clear(VISA resource name=w476, error in (no error)=w475) -> (VISA resource name out=w474:refnum<visa-resource-name>, error out=w473:errorcluster)
                  }
                  frame True {
                    n191 = Wait (ms)(milliseconds to wait=u32 100) -> ()  [unwired: 1 out]
                    n192 = VISA Read(VISA resource name=w483, byte count=u32 6, error in (no error)=w482) -> (VISA resource name out=w486:refnum<visa-resource-name>, read buffer=w478:string, error out=w485:errorcluster)  [unwired: 1 out]
                    n193 = Concatenate Strings(w479, w478) -> (w477:string)
                    n194 = local write item#1(w477) -> ()
                    n195 = call "Checksum.vi"("String"=w477, "Check soma?"=TRUE) -> ("Checksum?"=w484:bool)  [unwired: 1 in, 2 out]
                  }
                }
              }
              frame #3 {
                n196 = case shown="True" w488 {
                  tunnel: w488 -> [_ w492]
                  frame False {
                  }
                  frame True {
                    n197 = local write "Configurado Man"(w492) -> ()
                    n198 = local write "Configurado Auto"(FALSE ("Configurado Auto")) -> ()
                    "Configurado Man" <- w492
                  }
                }
              }
            }
          }
        }
      }
      frame "Start device" {
        n199 = local write "Pulso\nInstantâneo"(0 ("*(type *) &x")) -> ()
        n200 = Concatenate Strings("\nÀ" ("write buffer"), w494, "\u0003\u0000" ("write buffer")) -> (w497:string)
        n201 = call "Checksum.vi"("String"=w497) -> ("Checksum?"=w495:bool, "Check"=w496:string)  [unwired: 2 in, 1 out]
        n202 = Concatenate Strings(w497, w496, "\u000f" ("write buffer")) -> (w503:string)
        n203 = VISA Write(VISA resource name=w500, write buffer=w503, error in (no error)=w499) -> (VISA resource name out=w502:refnum<visa-resource-name>, error out=w501:errorcluster)  [unwired: 1 out]
        n204 = case shown="True" w495 {
          tunnel: [w510 w516] -> w508
          tunnel: [w509 w515] -> w507
          tunnel: [Control_1."erro" w512] -> w506
          tunnel: w502 -> [w510 w514]
          tunnel: w501 -> [w509 w513]
          frame False {
          }
          frame True {
            n205 = flat-sequence {
              tunnel: [w526] -> w522
              tunnel: [w525] -> w521
              tunnel: w514 -> [w524]
              tunnel: w513 -> [w523]
              tunnel: w522 -> [w534]
              tunnel: [w531] -> w520
              tunnel: w521 -> [w533]
              tunnel: [w530] -> w519
              tunnel: [w528] -> w518
              tunnel: [w527] -> w517
              tunnel: w520 -> [w541]
              tunnel: w519 -> [w540]
              tunnel: [w539] -> w516
              tunnel: [w538] -> w515
              tunnel: w518 -> [w537]
              tunnel: w517 -> [w536]
              tunnel: [Control_1."Wait"] -> w512
              frame #0 {
                n206 = property class="Instr" props=["Serial Settings:Number of Bytes at Serial Port"](reference=w524, error in=w523) -> (reference out=w526:refnum<visa-resource-name>, error out=w525:errorcluster)  [unwired: 1 out]
              }
              frame #1 {
                w527 = "\n" ("x")
                n207 = VISA Read(VISA resource name=w534, byte count=u32 1, error in (no error)=w533) -> (VISA resource name out=w531:refnum<visa-resource-name>, read buffer=w529:string, error out=w530:errorcluster)  [unwired: 1 out]
                n208 = Equal?(x=w527, y=w529) -> (x = y?=w528:bool)
              }
              frame #2 {
                n209 = case shown="True" w537 {
                  tunnel: w541 -> [w546 w556]
                  tunnel: w540 -> [w545 w555]
                  tunnel: [w544 w552] -> w539
                  tunnel: [w543 w551] -> w538
                  tunnel: w536 -> [_ w549]
                  frame False {
                    w542 = T3 16 items=["Flush Receive Buffer"=16, "Write Transmit Buffer to Device"=32, "Flush Receive Buffer (No I/O)"=64, "Flush Transmit Buffer"=128] ("Mask")
                    n210 = VISA Flush I/O Buffer(VISA resource name=w546, mask (16)=w542, error in (no error)=w545) -> (VISA resource name out=w544:refnum<visa-resource-name>, error out=w543:errorcluster)
                  }
                  frame True {
                    n211 = VISA Read(VISA resource name=w556, byte count=u32 6, error in (no error)=w555) -> (VISA resource name out=w552:refnum<visa-resource-name>, read buffer=w550:string, error out=w551:errorcluster)  [unwired: 1 out]
                    n212 = Concatenate Strings(w549, w550) -> (w548:string)
                    n213 = local write item#1(w548) -> ()
                    n214 = call "Checksum.vi"("String"=w548, "Check soma?"=TRUE) -> ("Checksum?"=w547:bool)  [unwired: 1 in, 2 out]
                    n215 = case shown="True" w547 {
                      selector: w547 -> [_ w558]
                      frame False {
                      }
                      frame True {
                        n216 = property on="Iniciar dispositivo" class="Bool"("DisabledEnum"=T2."Disabled and Grayed Out" ("Disabled")) -> ()  [unwired: 2 in, 2 out]
                        "start device" <- w558
                      }
                    }
                  }
                }
              }
            }
          }
        }
      }
      frame "Read Auto" {
        w563 = T2."Disabled" ("Disabled")
        w564 = T2."Disabled" ("Disabled")
        w586 = "\n" ("x")
        n217 = local read "iniicio"() -> (w578:u32)
        n218 = Tick Count (ms)() -> (millisecond timer value=w577:u32)
        n219 = Subtract(x=w577, y=w578) -> (x-y=w561:u32)
        n220 = property on="Limpar" class="Bool"("DisabledEnum"=w563) -> ()  [unwired: 2 in, 2 out]
        n221 = property on="Limpar" class="Bool"("DisabledEnum"=w564) -> ()  [unwired: 2 in, 2 out]
        n222 = property on="Codificar" class="Bool"("DisabledEnum"=w563) -> ()  [unwired: 2 in, 2 out]
        n223 = property on="Codificar" class="Bool"("DisabledEnum"=w564) -> ()  [unwired: 2 in, 2 out]
        n224 = property on="Identificar" class="Bool"("DisabledEnum"=w563) -> ()  [unwired: 2 in, 2 out]
        n225 = property on="Identificar" class="Bool"("DisabledEnum"=w564) -> ()  [unwired: 2 in, 2 out]
        n226 = property on="Inicia auto" class="Bool"("DisabledEnum"=w563) -> ()  [unwired: 2 in, 2 out]
        n227 = property on="Inicia auto" class="Bool"("DisabledEnum"=w564) -> ()  [unwired: 2 in, 2 out]
        n228 = Divide(x=w561, y=1000.0) -> (x/y=→"Tempo\nInstantâneo (ms)":dbl)
        n229 = Insert Into Array(array=w575, index=w576, new element=w561) -> (w574:u32[])
        n230 = property on="Iniciar dispositivo" class="Bool"("DisabledEnum"=w563) -> ()  [unwired: 2 in, 2 out]
        n231 = property on="Iniciar dispositivo" class="Bool"("DisabledEnum"=w564) -> ()  [unwired: 2 in, 2 out]
        n232 = property on="salvar dados" class="Bool"("DisabledEnum"=w563) -> ()  [unwired: 2 in, 2 out]
        n233 = property on="salvar dados" class="Bool"("DisabledEnum"=w564) -> ()  [unwired: 2 in, 2 out]
        n234 = property on="Configurar" class="Bool"("DisabledEnum"=w563) -> ()  [unwired: 2 in, 2 out]
        n235 = property on="Configurar" class="Bool"("DisabledEnum"=w564) -> ()  [unwired: 2 in, 2 out]
        n236 = Array Size(array=w574) -> ()  [unwired: 1 out]
        n237 = property class="Instr"(reference=w570, error in=w571) -> (reference out=w568:refnum<visa-resource-name>, error out=w569:errorcluster, "Serial Settings:Number of Bytes at Serial Port"=→"Serial Settings:Number of Bytes at Serial Port":u32)
        n238 = VISA Read(VISA resource name=w568, byte count=u32 1, error in (no error)=w569) -> (VISA resource name out=w588:refnum<visa-resource-name>, read buffer=w581:string, error out=w583:errorcluster)  [unwired: 1 out]
        n239 = Unbundle(w583) -> ("code"=w585:i32)  [unwired: 2 out]
        n240 = Equal?(x=w585, y=-1073807339) -> (x = y?=w582:bool)
        n241 = Equal?(x=w586, y=w581) -> (x = y?=w587:bool)
        n242 = Not(x=w582) -> (.not. x?=w580:bool)
        n243 = case shown="True" w580 {
          tunnel: [w600 w617] -> w590
          tunnel: [w599 w616] -> w589
          tunnel: w588 -> [w600 w615]
          tunnel: [w594 w611] -> w591
          tunnel: w583 -> [w601 w612]
          tunnel: w569 -> [w602 _]
          tunnel: w587 -> [_ w614]
          tunnel: w586 -> [_ w613]
          tunnel: w582 -> [w598 _]
          tunnel: [w593 w606] -> w579
          tunnel: w576 -> [w593 w610]
          tunnel: [w592 w609] -> w573
          tunnel: w572 -> [w592 w608]
          tunnel: [_ w605] -> w566
          tunnel: w565 -> [_ w603]
          frame False {
            n244 = Select(t=w602, s=w598, f=w601) -> (s? t:f=w599:errorcluster)
            n245 = local read "Parar"() -> (w597:bool)
            n246 = Select(t=Control_1."Stop device", s=w597, f=Control_1."Read Auto") -> (s? t:f=w594:T1)
          }
          frame True {
            n247 = flat-sequence {
              tunnel: [w629] -> w620
              tunnel: [w628] -> w619
              tunnel: [w627] -> w618
              tunnel: w615 -> [w626]
              tunnel: w614 -> [w625]
              tunnel: w613 -> [w624]
              tunnel: w612 -> [w623]
              tunnel: [w622] -> w607
              tunnel: w603 -> [w621]
              tunnel: [w621] -> w604
              tunnel: w620 -> [w673]
              tunnel: [w672] -> w616
              tunnel: w619 -> [w672]
              tunnel: [w673] -> w617
              tunnel: w618 -> [w653]
              tunnel: [w646] -> w611
              tunnel: w610 -> [w666]
              tunnel: [w665] -> w609
              tunnel: w608 -> [w664]
              tunnel: w607 -> [w663]
              tunnel: [w652] -> w606
              tunnel: [w651] -> w605
              tunnel: w604 -> [w650]
              frame #0 {
                n248 = case shown="True" w625 {
                  tunnel: w626 -> [w635 w645]
                  tunnel: w623 -> [w634 w644]
                  tunnel: [w633 w643] -> w629
                  tunnel: [w632 w642] -> w628
                  tunnel: [_ w638] -> w627
                  tunnel: w624 -> [_ w639]
                  tunnel: [FALSE ("Checksum?") w636] -> w622
                  frame False {
                    w631 = T3 16 items=["Flush Receive Buffer"=16, "Write Transmit Buffer to Device"=32, "Flush Receive Buffer (No I/O)"=64, "Flush Transmit Buffer"=128] ("Mask")
                    n249 = VISA Flush I/O Buffer(VISA resource name=w635, mask (16)=w631, error in (no error)=w634) -> (VISA resource name out=w633:refnum<visa-resource-name>, error out=w632:errorcluster)
                  }
                  frame True {
                    n250 = VISA Read(VISA resource name=w645, byte count=u32 66, error in (no error)=w644) -> (VISA resource name out=w643:refnum<visa-resource-name>, read buffer=w637:string, error out=w642:errorcluster)  [unwired: 1 out]
                    n251 = Concatenate Strings(w639, w637) -> (w638:string)
                    "?" <- w638
                    n252 = call "Checksum.vi"("String"=w638, "Check soma?"=TRUE) -> ("Checksum?"=w636:bool)  [unwired: 1 in, 2 out]
                  }
                }
              }
              frame #1 {
                w648 = Control_1."Stop device"
                n253 = case shown="True" w663 {
                  tunnel: w653 -> [_ w684]
                  tunnel: [TRUE FALSE] -> w667
                  tunnel: w666 -> [w678 w683]
                  tunnel: [w679 w687] -> w665
                  tunnel: w664 -> [w679 w686]
                  tunnel: [w678 w682] -> w652
                  tunnel: w650 -> [w677 w681]
                  tunnel: [w676 w681] -> w651
                  frame False {
                    n254 = Increment(x=w677) -> (x+1=w676:dbl)
                    "ERRO" <- w676
                  }
                  frame True {
                    n255 = Insert Into Array(array=w686, index=w683, new element=w684) -> (w687:string[])
                    n256 = Increment(x=w683) -> (x+1=w682:dbl)
                  }
                }
                n257 = String Subset(string=w653, offset (0)=5 ("length (rest)"), length (rest)=2 ("length (rest)")) -> (substring=w654:string)
                n258 = String Subset(string=w653, offset (0)=25 ("length (rest)"), length (rest)=4 ("length (rest)")) -> (substring=w662:string)
                n259 = local read "Configurado Man"() -> (w671:bool)
                n260 = Type Cast(type=u16 0, x=w654) -> ()  [unwired: 1 out]
                n261 = Type Cast(type=0, x=w662) -> (*(type *) &x=→"Pulso\nInstantâneo":i32)
                n262 = case shown="False" w671 {
                  tunnel: [Control_1."Read Auto" Control_1."Wait"] -> w670
                  frame False {
                  }
                  frame True {
                  }
                }
                n263 = local read "Parar"() -> (w647:bool)
                n264 = Select(t=w648, s=w647, f=w670) -> (s? t:f=w669:T1)
                n265 = Select(t=Control_1."Read Auto", s=w667, f=w669) -> (s? t:f=w649:T1)
                n266 = Select(t=w648, s=w647, f=w649) -> (s? t:f=w646:T1)
              }
            }
          }
        }
      }
      frame "Read Again" {
        n267 = Concatenate Strings("\nÀ" ("write buffer"), w694, "\u0005\u0000" ("write buffer")) -> (w703:string)
        n268 = call "Checksum.vi"("String"=w703, "Check soma?"=FALSE) -> ("Checksum?"=w696:bool, "Check"=w702:string)  [unwired: 1 in, 1 out]
        n269 = Concatenate Strings(w703, w702, "\u000f" ("write buffer")) -> (w700:string)
        n270 = VISA Write(VISA resource name=w690, write buffer=w700, error in (no error)=w689) -> (VISA resource name out=w699:refnum<visa-resource-name>, error out=w698:errorcluster)  [unwired: 1 out]
        n271 = case shown="True" w696 {
          tunnel: [w708 w712] -> w692
          tunnel: [w707 w711] -> w691
          tunnel: [Control_1."erro" Control_1."Read Auto"] -> w706
          tunnel: w699 -> [w708 w712]
          tunnel: w698 -> [w707 w711]
          frame False {
          }
          frame True {
          }
        }
      }
      frame "Read First" {
        n272 = flat-sequence {
          tunnel: w725 -> [w732]
          tunnel: w724 -> [w731]
          tunnel: w719 -> [w728]
          tunnel: [w730] -> w717
          tunnel: [w729] -> w716
          tunnel: w715 -> [_]
          tunnel: [w727] -> w714
          tunnel: [w742] -> w721
          tunnel: [w743] -> w722
          tunnel: [w744] -> w723
          tunnel: w717 -> [w744]
          tunnel: w716 -> [w743]
          tunnel: w714 -> [w742]
          frame #0 {
            n273 = Concatenate Strings("\nÀ" ("write buffer"), w728, "\u0004\u0000" ("write buffer")) -> (w735:string)
            n274 = call "Checksum.vi"("String"=w735, "Check soma?"=FALSE) -> ("Checksum?"=w726:bool, "Check"=w736:string)  [unwired: 1 in, 1 out]
            n275 = case shown="True" w726 {
              tunnel: [Control_1."erro" Control_1."Read Auto"] -> w727
              frame False {
              }
              frame True {
              }
            }
            n276 = Concatenate Strings(w735, w736, "\u000f" ("write buffer")) -> (w738:string)
            n277 = VISA Write(VISA resource name=w732, write buffer=w738, error in (no error)=w731) -> (VISA resource name out=w730:refnum<visa-resource-name>, error out=w729:errorcluster)  [unwired: 1 out]
          }
          frame #1 {
          }
        }
      }
      frame "Stop device" {
        n278 = flat-sequence {
          tunnel: w765 -> [w776]
          tunnel: w764 -> [w775]
          tunnel: [w774] -> w763
          tunnel: [w773] -> w762
          tunnel: w763 -> [w785]
          tunnel: w762 -> [w784]
          tunnel: [w783] -> w761
          tunnel: [w782] -> w760
          tunnel: w768 -> [w781]
          tunnel: [w798] -> w759
          tunnel: [w800] -> w758
          tunnel: [w799] -> w757
          tunnel: [w798] -> w751
          tunnel: w761 -> [w795]
          tunnel: w760 -> [w794]
          tunnel: [w806] -> w748
          tunnel: [w807] -> w749
          tunnel: [w805] -> w756
          tunnel: w759 -> [w804]
          tunnel: w758 -> [w803]
          tunnel: w757 -> [w802]
          frame #0 {
            n279 = property class="Instr"(reference=w776, error in=w775) -> (reference out=w777:refnum<visa-resource-name>, error out=w778:errorcluster, "Serial Settings:Number of Bytes at Serial Port"=w779:u32)
            n280 = Wait (ms)(milliseconds to wait=u32 100) -> ()  [unwired: 1 out]
            n281 = VISA Read(VISA resource name=w777, byte count=w779, error in (no error)=w778) -> (VISA resource name out=w774:refnum<visa-resource-name>, error out=w773:errorcluster)  [unwired: 2 out]
          }
          frame #1 {
            (unwired) FALSE ("Checksum?")
            n282 = Wait (ms)(milliseconds to wait=u32 100) -> ()  [unwired: 1 out]
            n283 = Concatenate Strings("\nÀ" ("write buffer"), w781, "\u0006\u0000" ("write buffer")) -> (w789:string)
            n284 = call "Checksum.vi"("String"=w789, "Check soma?"=FALSE) -> ("Check"=w788:string)  [unwired: 1 in, 2 out]
            n285 = Concatenate Strings(w789, w788, "\u000f" ("write buffer")) -> (w792:string)
            n286 = VISA Write(VISA resource name=w785, write buffer=w792, error in (no error)=w784) -> (VISA resource name out=w783:refnum<visa-resource-name>, error out=w782:errorcluster)  [unwired: 1 out]
          }
          frame #2 {
            n287 = Wait (ms)(milliseconds to wait=u32 100) -> ()  [unwired: 1 out]
            n288 = VISA Read(VISA resource name=w795, byte count=u32 1, error in (no error)=w794) -> (VISA resource name out=w800:refnum<visa-resource-name>, read buffer=w797:string, error out=w799:errorcluster)  [unwired: 1 out]
            n289 = local write item#1(w797) -> ()
            n290 = Equal?(x="\n", y=w797) -> (x = y?=w798:bool)
          }
          frame #3 {
            n291 = case shown="False" w804 {
              tunnel: [w809 w820] -> w807
              tunnel: [w808 w819] -> w806
              tunnel: [FALSE ("Checksum?") w818] -> w805
              tunnel: w803 -> [w809 w816]
              tunnel: w802 -> [w808 w815]
              frame False {
              }
              frame True {
                n292 = VISA Read(VISA resource name=w816, byte count=u32 6, error in (no error)=w815) -> (VISA resource name out=w814:refnum<visa-resource-name>, read buffer=w812:string, error out=w813:errorcluster)  [unwired: 1 out]
                n293 = Concatenate Strings("\n" ("string"), w812) -> (w821:string)
                n294 = local write item#1(w821) -> ()
                n295 = call "Checksum.vi"("String"=w821, "Check soma?"=TRUE) -> ("Checksum?"=w818:bool)  [unwired: 1 in, 2 out]
                n296 = case shown="False" w818 {
                  tunnel: [w825 w829] -> w820
                  tunnel: [w826 w828] -> w819
                  tunnel: w814 -> [w824 w829]
                  tunnel: w813 -> [w823 w828]
                  frame False {
                    n297 = VISA Clear(VISA resource name=w824, error in (no error)=w823) -> (VISA resource name out=w825:refnum<visa-resource-name>, error out=w826:errorcluster)
                  }
                  frame True {
                    n298 = local write "save"(FALSE ("save")) -> ()
                    n299 = local write "start read"(FALSE ("start read")) -> ()
                    n300 = local write "start device"(FALSE ("start device")) -> ()
                    n301 = property on="Inicia auto" class="Bool"("DisabledEnum"=T2."Enabled" ("Disabled")) -> ()  [unwired: 2 in, 2 out]
                  }
                }
              }
            }
          }
        }
        n302 = local write "Parar"(FALSE ("Parar")) -> ()
        n303 = Select(t=Control_1."Organize", s=w751, f=Control_1."Stop device") -> (s? t:f=w754:T1)
        n304 = property class="Instr"(reference=w749, error in=w748) -> (reference out=w747:refnum<visa-resource-name>, error out=w746:errorcluster, "Serial Settings:Number of Bytes at Serial Port"=w745:u32)
        n305 = Select(t=w754, s=w756, f=Control_1."Stop device") -> (s? t:f=w769:T1)
        n306 = VISA Read(VISA resource name=w747, byte count=w745, error in (no error)=w746) -> (VISA resource name out=w770:refnum<visa-resource-name>, error out=w771:errorcluster)  [unwired: 2 out]
      }
      frame "End" {
        (unwired) TRUE
        n307 = local write "stop"(FALSE ("start device")) -> ()
      }
      frame "Save" {
        n308 = call-poly <vilib>:"Write Delimited Spreadsheet.vi"("1D data"=w849, "append to file? (new file:F)"=TRUE, "transpose? (no:F)"=FALSE) -> ("new file path (Not A Path if cancelled)"=w846:path, "error out"=w848:errorcluster)  [unwired: 11 in]
        n309 = Unbundle(w848) -> ("status"=w847:bool)  [unwired: 2 out]
        n310 = case shown="False" w847 {
          tunnel: w846 -> [w857 _]
          tunnel: w845 -> [w855 _]
          tunnel: [w858 TRUE ("status")] -> w844
          tunnel: w840 -> [w856 _]
          tunnel: w839 -> [w854 _]
          tunnel: w838 -> [w853 _]
          frame False {
            n311 = Build Array(w856, w854, w855, w853) -> (w862:string[][])
            n312 = call-poly <vilib>:"Write Delimited Spreadsheet.vi"("file path (dialog if empty)"=w857, "2D data"=w862, "append to file? (new file:F)"=TRUE, "transpose? (no:F)"=TRUE) -> ("error out"=w859:errorcluster)  [unwired: 10 in, 1 out]
            n313 = Unbundle(w859) -> ("status"=w858:bool)  [unwired: 2 out]
          }
          frame True {
          }
        }
        n314 = case shown="False" w844 {
          frame False {
            "save" <- TRUE ("salvar dados")
          }
          frame True {
          }
        }
      }
      frame "Organize" {
        n315 = while {
          tunnel: w874 -> [w897] mode=indexing
          tunnel: w873 -> [w886]
          shift-right: [w895] -> _
          shift-left: w867 -> [w896]
          shift-right: [w885] -> w872
          shift-left: w871 -> [w884]
          shift-right: [w883] -> w870
          shift-left: w866 -> [w879]
          shift-right: [w881] -> w869
          shift-left: w865 -> [w880]
          shift-right: [w882] -> w868
          shift-left: w864 -> [w878]
          i -> [w893]
          stop <- w888 stop-if-true
          n316 = Equal?(x=0.0, y=w886) -> (x = y?=w889:bool)
          n317 = while {
            tunnel: w897 -> [w930]
            shift-right: [w917] -> w895
            shift-left: w896 -> [w910]
            shift-right: [w928] -> _
            shift-left: 3 ("y") -> [w920]
            shift-right: [w925] -> _
            shift-left: 21 ("y") -> [w919]
            shift-right: [w921] -> _
            shift-left: 0.0 -> [w922]
            shift-right: [w902] -> w882
            shift-left: w878 -> [w907]
            shift-right: [w909] -> w881
            shift-left: w880 -> [w906]
            shift-right: [w903] -> w883
            shift-left: w879 -> [w905]
            shift-right: [w908] -> w885
            shift-left: w884 -> [w904]
            stop <- w924 stop-if-true
            n318 = Increment(x=w922) -> (x+1=w921:dbl)
            n319 = Increment(x=w910) -> (x+1=w917:dbl)
            n320 = Add(x=w920, y=2) -> (x+y=w928:i32)
            n321 = Add(x=w919, y=4) -> (x+y=w925:i32)
            n322 = Number To Decimal String(number=w917) -> (decimal integer string=w913:string)  [unwired: 1 in]
            n323 = Equal?(x=1.0, y=w917) -> (x = y?=w918:bool)
            n324 = String Subset(string=w930, offset (0)=w925, length (rest)=4 ("length (rest)")) -> (substring=w932:string)
            n325 = String Subset(string=w930, offset (0)=w928, length (rest)=2 ("length (rest)")) -> (substring=w931:string)
            n326 = Equal?(x=w921, y=10.0) -> (x = y?=w924:bool)
            n327 = case shown="True" w918 {
              tunnel: ["" ("RingText.Text") w938] -> w914
              frame False {
              }
              frame True {
                n328 = local read "Configurado Auto"() -> (w939:bool)
                n329 = case shown="True" w939 {
                  tunnel: [w940 w942] -> w938
                  frame False {
                    n330 = local read "Frequência \nManual (Hz)"() -> (w941:i16)
                    n331 = Number To Decimal String(number=w941) -> (decimal integer string=w940:string)  [unwired: 1 in]
                  }
                  frame True {
                    n332 = property on="Frequência \nAutomática (Hz)" class="Ring (strict)"() -> ("RingText.Text"=w942:string)  [unwired: 2 in, 2 out]
                  }
                }
              }
            }
            n333 = Insert Into Array(array=w907, index=w910, new element=w913) -> (w902:string[])
            n334 = Type Cast(type=0, x=w932) -> (*(type *) &x=w915:i32)
            n335 = Type Cast(type=u16 0, x=w931) -> (*(type *) &x=w929:u16)
            n336 = Number To Decimal String(number=w915) -> (decimal integer string=w911:string)  [unwired: 1 in]
            n337 = Number To Decimal String(number=w929) -> (decimal integer string=w912:string)  [unwired: 1 in]
            n338 = Insert Into Array(array=w904, index=w910, new element=w911) -> (w908:string[])
            n339 = Insert Into Array(array=w905, index=w910, new element=w912) -> (w903:string[])
            n340 = Insert Into Array(array=w906, index=w910, new element=w914) -> (w909:string[])
          }
          n341 = Increment(x=w893) -> (x+1=w887:i32)
          n342 = case shown="False" w889 {
            tunnel: [w898 TRUE] -> w888
            tunnel: w887 -> [w900 _]
            tunnel: w886 -> [w899 _]
            frame False {
              n343 = Equal?(x=w900, y=w899) -> (x = y?=w898:bool)
            }
            frame True {
            }
          }
        }
      }
      frame "erro" {
        n344 = flat-sequence {
          tunnel: w951 -> [w956]
          tunnel: w950 -> [w957]
          tunnel: [w955] -> w949
          tunnel: [w954] -> w948
          tunnel: [w953] -> w947
          tunnel: [w952] -> w946
          tunnel: w949 -> [w966]
          tunnel: w948 -> [w965]
          tunnel: w947 -> [w964]
          tunnel: w946 -> [w963]
          tunnel: [w962] -> w945
          tunnel: [w961] -> w944
          tunnel: [w960] -> w943
          frame #0 {
            w952 = "\n" ("x")
            n345 = VISA Read(VISA resource name=w957, byte count=u32 1, error in (no error)=w956) -> (VISA resource name out=w954:refnum<visa-resource-name>, read buffer=w958:string, error out=w955:errorcluster)  [unwired: 1 out]
            n346 = local write item#1(w958) -> ()
            n347 = Equal?(x=w952, y=w958) -> (x = y?=w953:bool)
          }
          frame #1 {
            n348 = case shown="False" w964 {
              tunnel: w965 -> [w972 w983]
              tunnel: w966 -> [w971 w982]
              tunnel: [w970 w979] -> w962
              tunnel: [w969 w978] -> w961
              tunnel: w963 -> [_ w976]
              tunnel: [Control_1."Wait" w973] -> w960
              frame False {
                w968 = T3 16 items=["Flush Receive Buffer"=16, "Write Transmit Buffer to Device"=32, "Flush Receive Buffer (No I/O)"=64, "Flush Transmit Buffer"=128] ("Mask")
                n349 = VISA Flush I/O Buffer(VISA resource name=w972, mask (16)=w968, error in (no error)=w971) -> (VISA resource name out=w970:refnum<visa-resource-name>, error out=w969:errorcluster)
              }
              frame True {
                n350 = VISA Read(VISA resource name=w983, byte count=u32 7, error in (no error)=w982) -> (VISA resource name out=w979:refnum<visa-resource-name>, read buffer=w977:string, error out=w978:errorcluster)  [unwired: 1 out]
                n351 = Concatenate Strings(w976, w977) -> (w975:string)
                n352 = local write item#1(w975) -> ()
                n353 = call "Checksum.vi"("String"=w975, "Check soma?"=TRUE) -> ("Checksum?"=w974:bool)  [unwired: 1 in, 2 out]
                n354 = case shown="True" w974 {
                  tunnel: [Control_1."Wait" Control_1."Wait"] -> w973
                  frame False {
                  }
                  frame True {
                  }
                }
              }
            }
          }
        }
      }
      frame "Plot" {
        n355 = Array Size(array=w990) -> (size(s)=w997:i32)
        n356 = for {
          N: w997 -> [_]
          tunnel: w990 -> [w1002] mode=indexing
          shift-right: [w999] -> w995
          shift-left: i32[] [] -> [w998]
          i -> [w1000]
          n357 = Decimal String To Number(string=w1002) -> (number=w1001:i32)  [unwired: 2 in, 1 out]
          n358 = Insert Into Array(array=w998, index=w1000, new element=w1001) -> (w999:i32[])
        }
        n359 = Bundle By Name("Y"=w995, "dt"=1.0) -> (→"Waveform Graph":waveform(i32))  [unwired: 1 in]
      }
    }
    n360 = Unbundle(w55) -> ("status"=w54:bool)  [unwired: 2 out]
    n361 = local read "stop"() -> (w41:bool)
    n362 = Or(x=w41, y=w54) -> (x .or. y?=w53:bool)
    n363 = case shown="True" w53 {
      tunnel: w61 -> [w66 w73]
      tunnel: w55 -> [w65 w72]
      tunnel: [w66 _] -> w60
      tunnel: [w65 w68] -> w59
      frame False {
      }
      frame True {
        w67 = FALSE ("Configurado Man")
        w70 = T3 128 items=["Flush Receive Buffer"=16, "Write Transmit Buffer to Device"=32, "Flush Receive Buffer (No I/O)"=64, "Flush Transmit Buffer"=128] ("Mask")
        n364 = local write "stop"(w67) -> ()
        n365 = local write "Configurado Man"(w67) -> ()
        n366 = local write "Configurado Auto"(w67) -> ()
        n367 = local write "Conectado"(w67) -> ()
        n368 = VISA Flush I/O Buffer(VISA resource name=w73, mask (16)=w70, error in (no error)=w72) -> (VISA resource name out=w71:refnum<visa-resource-name>, error out=w69:errorcluster)
        n369 = VISA Close(VISA resource name=w71, error in (no error)=w69) -> (error out=w68:errorcluster)
      }
    }
  }
